vi "SA5G_setEVMDemodulation.vi"(7 "Func":enum16{"Low", "High"}(ring), 8 "error in":errorcluster, 11 "VISA in":refnum<visa-resource-name>) -> (0 "error out":errorcluster, 2 "SA_Resp":string, 3 "VISA out":refnum<visa-resource-name>)   [LabVIEW 2023, in "Keysight.lvlib"]
uses:
  Keysight.lvlib
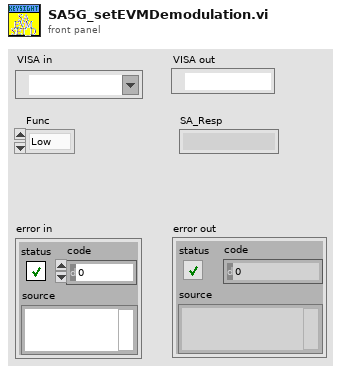
[diagram p1: front panel]
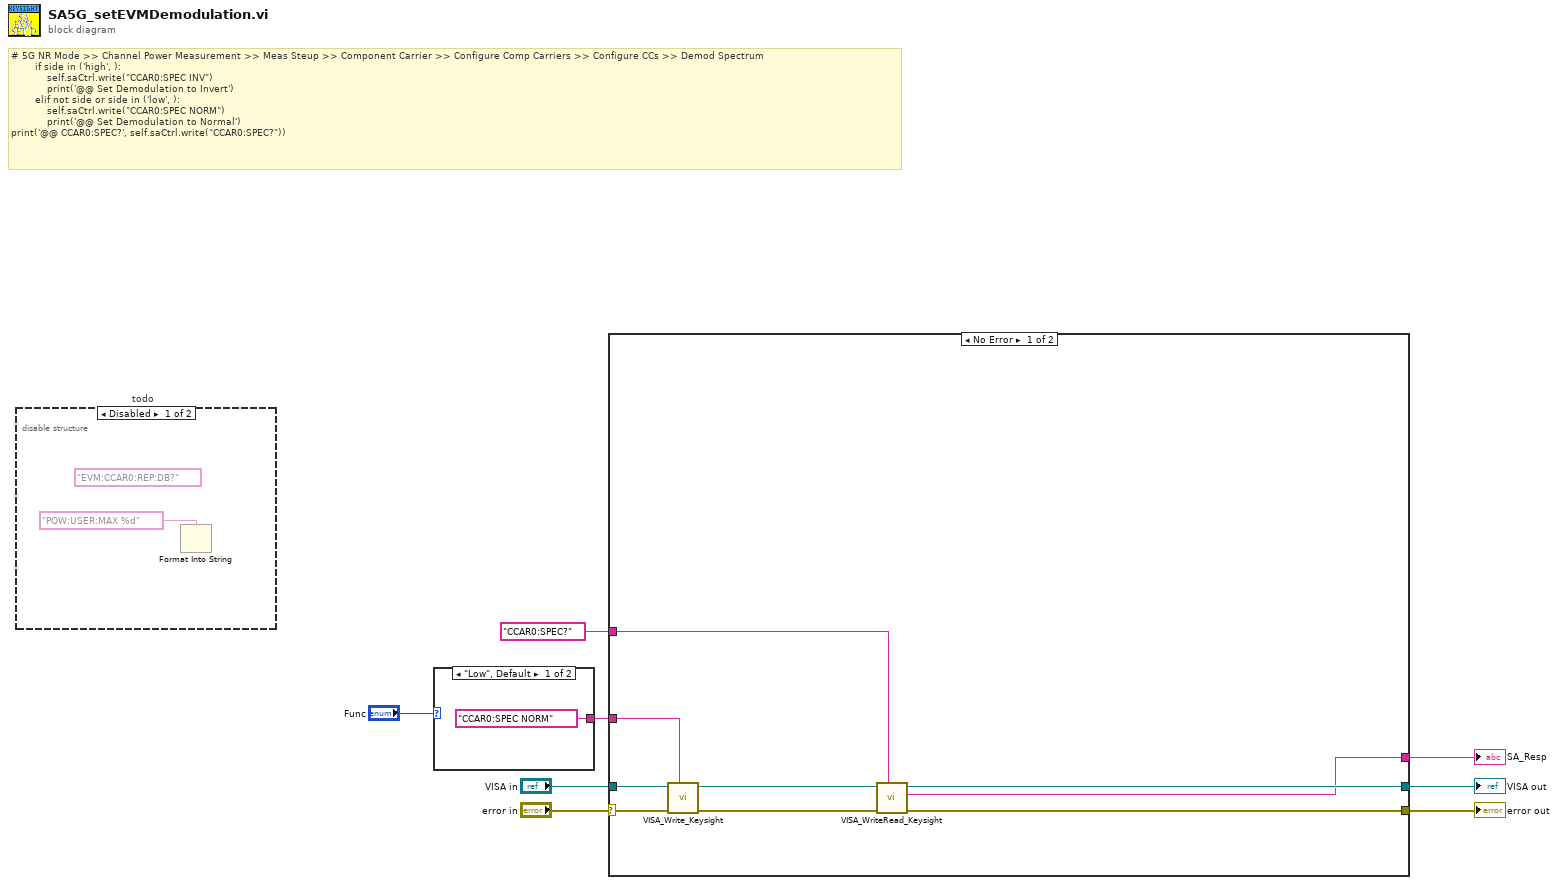
[diagram p0: block diagram]
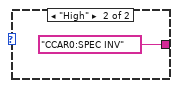
[diagram p2: hidden frame]
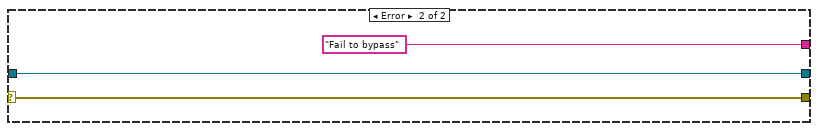
[diagram p4: hidden frame]
diagram:
  # "# 5G NR Mode >> Channel Power Measurement >> Meas Steup >> Component Carrier >> Configure Comp Carriers >> Configure CCs >> Demod Spectrum\n        if side in ('high', ):\n            self.saCtrl.write(\"CCAR0:SPEC INV\")\n            print('@@ Set Demodulation to Invert')\n        elif not side or side in ('low', ):\n            self.saCtrl.write(\"CCAR0:SPEC NORM\")\n            print('@@ Set Demodulation to Normal')\nprint('@@ CCAR0:SPEC?', self.saCtrl.write(\"CCAR0:SPEC?\"))"
  n1 = disable-structure "todo" shown="Disabled" {
    frame Disabled {
      (unwired) "EVM:CCAR0:REP:DB?" ("write buffer")
      n2 = Format Into String(format string="POW:USER:MAX %d") -> ()  [unwired: 3 in, 2 out]
    }
    frame Enabled {
    }
  }
  n3 = case shown="\"Low\", Default" "Func" {
    tunnel: ["CCAR0:SPEC NORM" ("write buffer") "CCAR0:SPEC INV" ("write buffer")] -> w8
    frame "Low", Default {
    }
    frame "High" {
    }
  }
  n4 = case shown="No Error" "error in" {
    selector: "error in" -> [w20 w22]
    tunnel: "VISA in" -> [w19 w23]
    tunnel: w8 -> [w18 _]
    tunnel: [w17 w22] -> w5
    tunnel: [w16 w23] -> w6
    tunnel: [w15 "Fail to bypass" ("Response")] -> w7
    tunnel: "CCAR0:SPEC?" ("write buffer") -> [w12 _]
    frame No Error {
      n5 = call "VISA_Write_Keysight.vi"("VISA CMD"=w18, "error in"=w20, "VISA in"=w19) -> ("error out"=w13:errorcluster, "VISA out"=w14:refnum<visa-resource-name>)  [unwired: 7 in]
      n6 = call "VISA_WriteRead_Keysight.vi"("VISA_CMD"=w12, "error in"=w13, "VISA in"=w14) -> ("error out"=w17:errorcluster, "Response"=w15:string, "VISA out"=w16:refnum<visa-resource-name>)  [unwired: 6 in]
    }
    frame Error {
    }
  }
  "SA_Resp" <- w7
  "VISA out" <- w6
  "error out" <- w5
